vi "Query Stored Values.vi"(8 "error in (no error)":errorcluster, 11 "VISA resource name":refnum<visa-resource-name>) -> (0 "error out":errorcluster, 1 "Minimum":dbl format="%#_10g", 2 "Maximum":dbl format="%#_10g", 3 "VISA resource name out":refnum<visa-resource-name>, 4 "Frequency":dbl format="%#_10g", 5 "Peak to Peak":dbl format="%#_10g")   [LabVIEW 2011, in "Fluke 8508.lvlib"]
doc: "This VI queries the Frequency(of the most recently triggered measurement), Minimum, Maximum, and Peak to Peak values on the instrument."
uses:
  Fluke 8508.lvlib
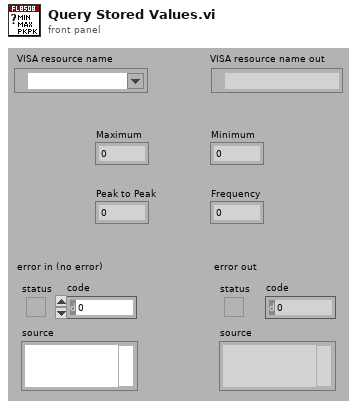
[diagram p1: front panel]
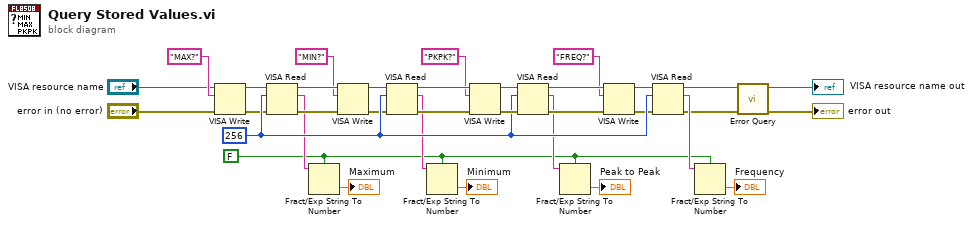
[diagram p0: block diagram]
diagram:
  w3 = FALSE ("use system decimal point (T)")
  w32 = u32 256 ("byte count")
  n1 = VISA Write(VISA resource name="VISA resource name", write buffer="MAX?", error in (no error)="error in (no error)") -> (VISA resource name out=w31:refnum<visa-resource-name>, error out=w30:errorcluster)  [unwired: 1 out]
  n2 = VISA Read(VISA resource name=w31, byte count=w32, error in (no error)=w30) -> (VISA resource name out=w29:refnum<visa-resource-name>, read buffer=w18:string, error out=w28:errorcluster)  [unwired: 1 out]
  n3 = Fract/Exp String To Number(use system decimal point (T)=w3, string=w18) -> (number=→"Maximum":dbl)  [unwired: 2 in, 1 out]
  n4 = VISA Write(VISA resource name=w29, write buffer="MIN?", error in (no error)=w28) -> (VISA resource name out=w27:refnum<visa-resource-name>, error out=w26:errorcluster)  [unwired: 1 out]
  n5 = VISA Read(VISA resource name=w27, byte count=w32, error in (no error)=w26) -> (VISA resource name out=w25:refnum<visa-resource-name>, read buffer=w15:string, error out=w24:errorcluster)  [unwired: 1 out]
  n6 = Fract/Exp String To Number(use system decimal point (T)=w3, string=w15) -> (number=→"Minimum":dbl)  [unwired: 2 in, 1 out]
  n7 = VISA Write(VISA resource name=w25, write buffer="PKPK?", error in (no error)=w24) -> (VISA resource name out=w33:refnum<visa-resource-name>, error out=w34:errorcluster)  [unwired: 1 out]
  n8 = VISA Read(VISA resource name=w33, byte count=w32, error in (no error)=w34) -> (VISA resource name out=w23:refnum<visa-resource-name>, read buffer=w13:string, error out=w22:errorcluster)  [unwired: 1 out]
  n9 = Fract/Exp String To Number(use system decimal point (T)=w3, string=w13) -> (number=→"Peak to Peak":dbl)  [unwired: 2 in, 1 out]
  n10 = VISA Write(VISA resource name=w23, write buffer="FREQ?", error in (no error)=w22) -> (VISA resource name out=w20:refnum<visa-resource-name>, error out=w21:errorcluster)  [unwired: 1 out]
  n11 = VISA Read(VISA resource name=w20, byte count=w32, error in (no error)=w21) -> (VISA resource name out=w5:refnum<visa-resource-name>, read buffer=w11:string, error out=w7:errorcluster)  [unwired: 1 out]
  n12 = Fract/Exp String To Number(use system decimal point (T)=w3, string=w11) -> (number=→"Frequency":dbl)  [unwired: 2 in, 1 out]
  n13 = call "Error Query.vi"("error in (no error)"=w7, "VISA resource name"=w5) -> ("error out"=→"error out":errorcluster, "VISA resource name out"=→"VISA resource name out":refnum<visa-resource-name>)  [unwired: 6 in, 2 out]
